vi "temperature_controller.vi"() -> ()   [LabVIEW 2017]
doc: "Use this template to build a simple state machine design pattern. Each state executes code and determines which state to transition to."
uses:
  controls/State.ctl
  <vilib>/Utility/error.llb/DialogType.ctl
  <instrlib>/LakeShore 336/Public/Data/Sensor Data (Single Reading).vi
  <instrlib>/LakeShore 336/Lake Shore 336.lvlib
panel:
  out "SetPoint":dbl format="%#_5f"
  out "Session Out":refnum<visa-resource-name>
  out "error out":errorcluster
  in  "Session In":refnum<visa-resource-name>="LakeShore336"
  in  "error in (no error)":errorcluster
  in  "SetPoint":dbl
  out "Heater percent":dbl
  in  "Heater":u16(ring) items=["Off", "Low", "Medium", "High"]
  out "Input A":dbl format="%#_5f"
  out "Input B":dbl format="%#_5f"
  in  "Exit Button":bool
  out "Status":string="Shutting down..."
  # "K"
  # "K"
  # "%"
  # "K"
  # "K"
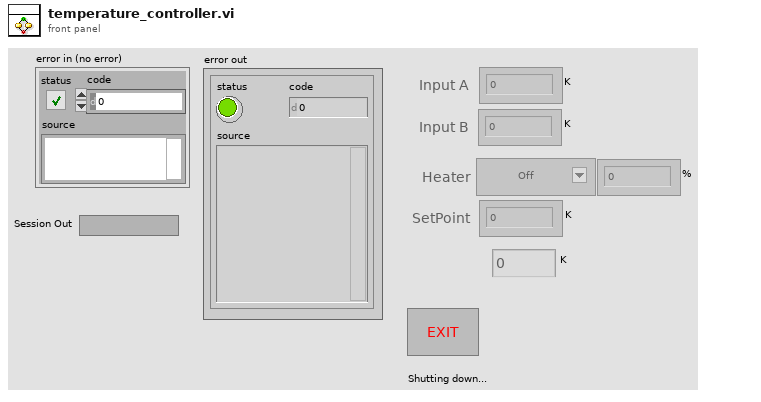
[diagram p1: front panel]
types:
  T1 = typedef "State.ctl" = enum16{"Init", "Idle", "Shutdown"}
  T2 = cluster{"Baud Rate":u32, "Parity":u16, "Data Bits":u16, "Stop Bits":u16, "Flow Control":u16}
  T3 = typedef "DialogType.ctl" = u16
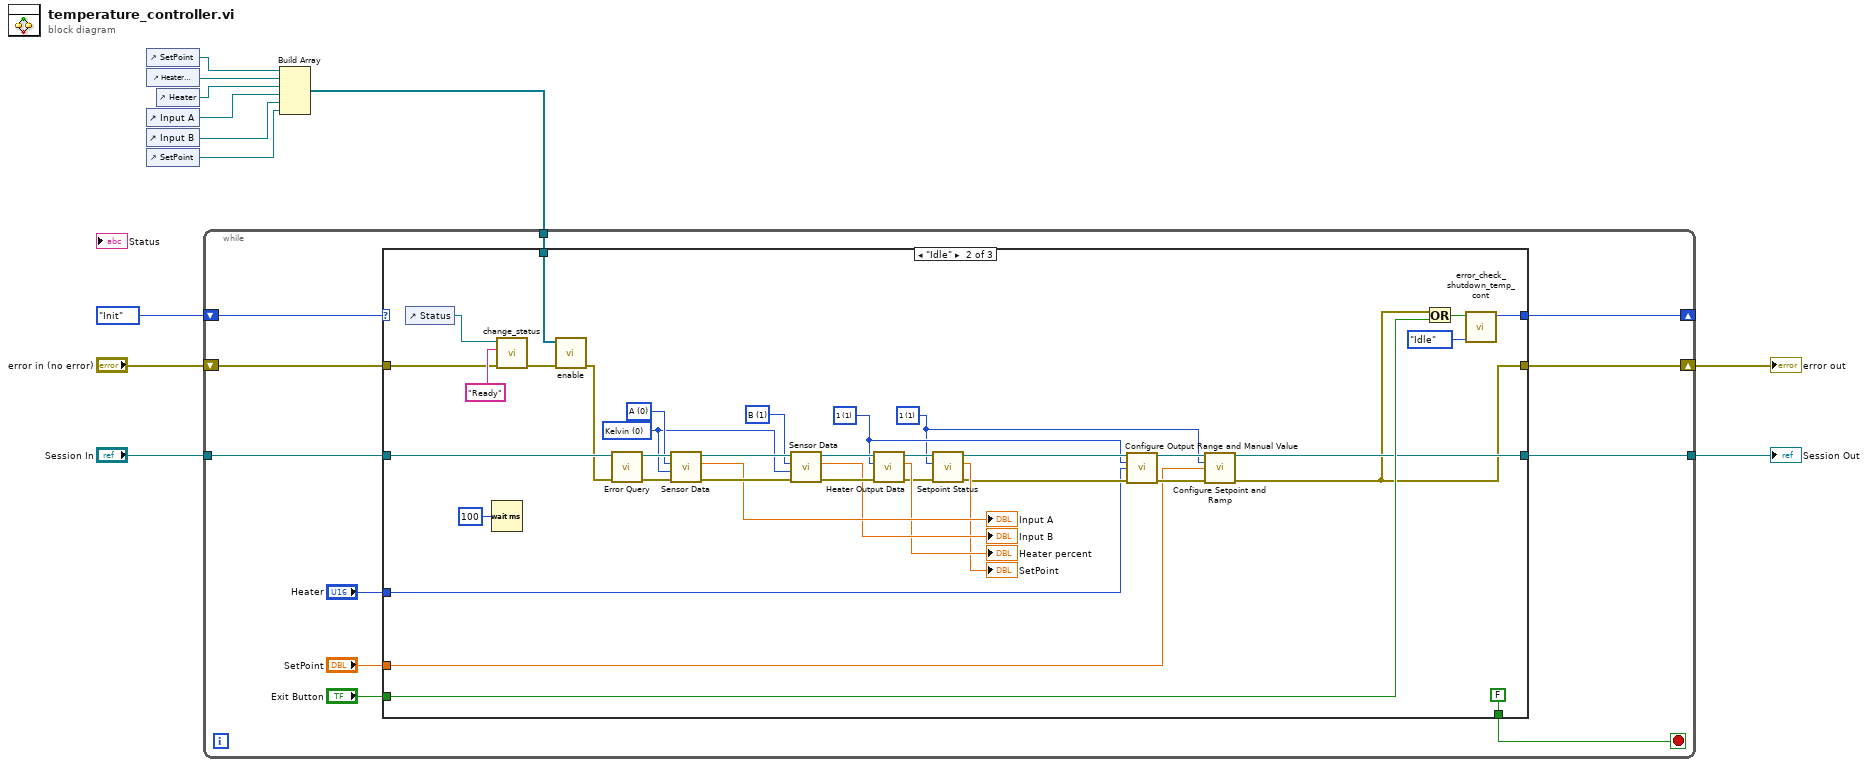
[diagram p0: block diagram]
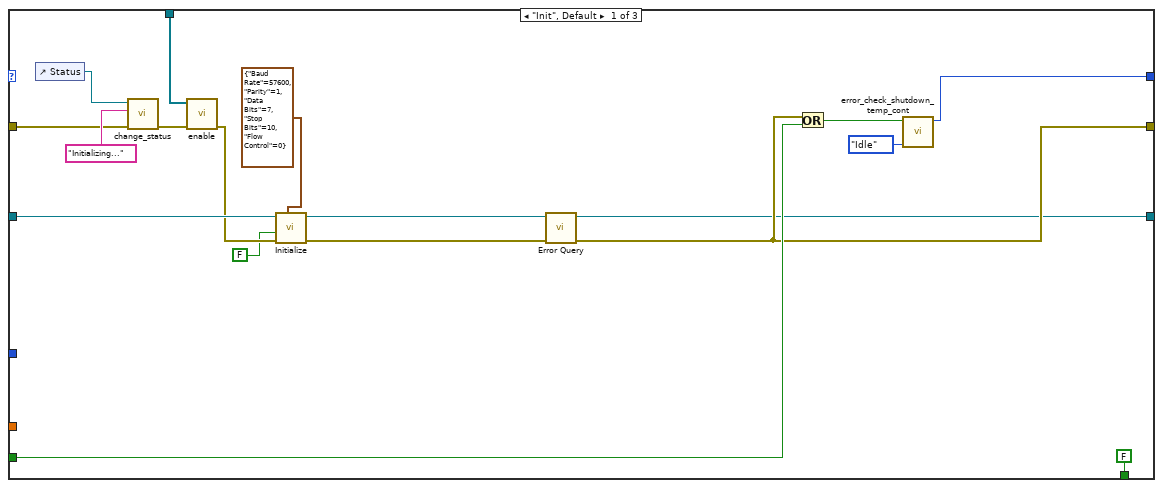
[diagram p2: hidden frame]
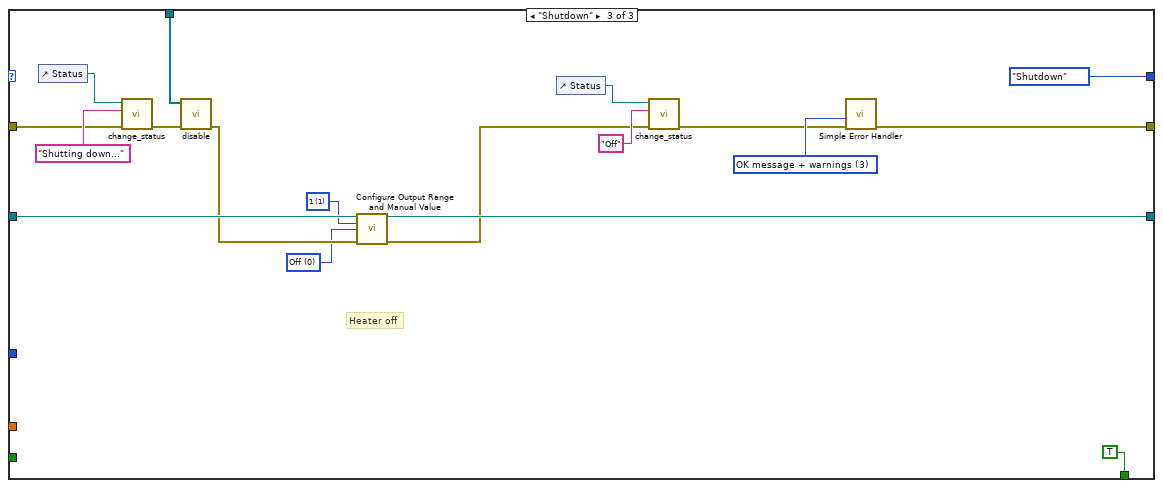
[diagram p3: hidden frame]
diagram:
  n1 = control-ref of="SetPoint"() -> (w12:refnum<vi>)
  n2 = control-ref of="Heater percent"() -> (w11:refnum<vi>)
  n3 = control-ref of="Input A"() -> (w9:refnum<vi>)
  n4 = control-ref of="Input B"() -> (w8:refnum<vi>)
  n5 = control-ref of="SetPoint"() -> (w1:refnum<vi>)
  n6 = control-ref of="Heater"() -> (w10:refnum<vi>)
  n7 = Build Array(w12, w11, w10, w9, w8, w1) -> (w7:refnum<vi>[])
  n8 = while {
    tunnel: w7 -> [w23]
    shift-right: [w18] -> _
    shift-left: State."Init" ("States") -> [w22]
    tunnel: "Session In" -> [w20]
    shift-right: [w19] -> w3
    shift-left: "error in (no error)" -> [w21]
    tunnel: [w14] -> w2
    stop <- w13 stop-if-true
    n9 = case shown="\"Idle\"" w22 {
      tunnel: w23 -> [w37 w79 w94]
      tunnel: w21 -> [w39 w75 w95]
      tunnel: w20 -> [w31 w68 w85]
      tunnel: [w29 w42 w92] -> w19
      tunnel: [w33 w71 State."Shutdown" ("s? t:f")] -> w18
      tunnel: "Exit Button" -> [w36 w72 _]
      tunnel: "Heater" -> [_ w48 _]
      tunnel: "SetPoint" -> [_ w44 _]
      tunnel: [w28 w45 w84] -> w14
      tunnel: [FALSE FALSE TRUE] -> w13
      frame "Init", Default {
        n10 = control-ref of="Status"() -> (w38:refnum<vi>)
        n11 = call "change_status.vi"("error in (no error)"=w39, "String"="Initializing...", "String in"=w38) -> ("error out"=w41:errorcluster)  [unwired: 8 in]
        n12 = call "enable.vi"("error in (no error)"=w41, "Array"=w37) -> ("error out"=w30:errorcluster)  [unwired: 9 in]
        n13 = call <instrlib>:"Initialize.vi"("Serial Configuration"=T2 {"Baud Rate"=57600, "Parity"=1, "Data Bits"=7, "Stop Bits"=10, "Flow Control"=0}, "error in (no error)"=w30, "Reset (True)"=FALSE, "VISA resource name"=w31) -> ("error out"=w24:errorcluster, "VISA resource name out"=w25:refnum<visa-resource-name>)  [unwired: 6 in]
        n14 = call <instrlib>:"Error Query.vi"("error in (no error)"=w24, "VISA resource name"=w25) -> ("error out"=w29:errorcluster, "VISA resource name out"=w28:refnum<visa-resource-name>)  [unwired: 7 in, 1 out]
        n15 = Or(x=w29, y=w36) -> (x .or. y?=w35:bool)
        n16 = call "error_check_shutdown_temp_cont.vi"("f"=State."Idle", "Boolean"=w35) -> ("s? t:f"=w33:T1)  [unwired: 9 in]
      }
      frame "Idle" {
        w43 = u16 1 items=["1"=1, "2"=2, "3"=3, "4"=4] ("Output (1:1)")
        w49 = u16 1 items=["1"=1, "2"=2] ("Heater Output (1:1)")
        w61 = u16 1 items=["A", "B", "C", "D"] ("Input (0:A)")
        w60 = u16 0 items=["Kelvin", "Celsius", "Sensor Units"] ("Data Source (0:Kelvin)")
        w64 = u16 0 items=["A", "B", "C", "D"] ("Input (0:A)")
        n17 = control-ref of="Status"() -> (w77:refnum<vi>)
        n18 = Wait (ms)(milliseconds to wait=u32 100) -> ()  [unwired: 1 out]
        n19 = call "change_status.vi"("error in (no error)"=w75, "String"="Ready", "String in"=w77) -> ("error out"=w78:errorcluster)  [unwired: 8 in]
        n20 = call "enable.vi"("error in (no error)"=w78, "Array"=w79) -> ("error out"=w67:errorcluster)  [unwired: 9 in]
        n21 = call <instrlib>:"Error Query.vi"("error in (no error)"=w67, "VISA resource name"=w68) -> ("error out"=w65:errorcluster, "VISA resource name out"=w66:refnum<visa-resource-name>)  [unwired: 7 in, 1 out]
        n22 = call-poly <instrlib>:"Sensor Data.vi"("error in (no error)"=w65, "Data Source (0:Kelvin)"=w60, "Input (0:A)"=w64, "VISA resource name"=w66) -> ("error out"=w62:errorcluster, "Sensor Data"=→"Input A":dbl, "VISA resource name out"=w63:refnum<visa-resource-name>)  [unwired: 5 in]
        n23 = call-poly <instrlib>:"Sensor Data.vi"("error in (no error)"=w62, "Data Source (0:Kelvin)"=w60, "Input (0:A)"=w61, "VISA resource name"=w63) -> ("error out"=w58:errorcluster, "Sensor Data"=→"Input B":dbl, "VISA resource name out"=w59:refnum<visa-resource-name>)  [unwired: 5 in]
        n24 = call <instrlib>:"Heater Output Data.vi"("error in (no error)"=w58, "Heater Output (1:1)"=w49, "VISA resource name"=w59) -> ("error out"=w53:errorcluster, "Output Value"=→"Heater percent":dbl, "VISA resource name out"=w54:refnum<visa-resource-name>)  [unwired: 6 in]
        n25 = call <instrlib>:"Setpoint Status.vi"("error in (no error)"=w53, "Output (1:1)"=w43, "VISA resource name"=w54) -> ("error out"=w50:errorcluster, "Setpoint"=→"SetPoint":dbl, "VISA resource name out"=w51:refnum<visa-resource-name>)  [unwired: 6 in]
        n26 = call <instrlib>:"Configure Output Range and Manual Value.vi"("VISA resource name"=w51, "Output (1:1)"=w49, "Range (0:Off)"=w48, "error in (no error)"=w50) -> ("VISA resource name out"=w47:refnum<visa-resource-name>, "error out"=w46:errorcluster)  [unwired: 10 in]
        n27 = call <instrlib>:"Configure Setpoint and Ramp.vi"("VISA resource name"=w47, "Output's Control Loop (1:1)"=w43, "Setpoint (0.00000)"=w44, "error in (no error)"=w46) -> ("VISA resource name out"=w45:refnum<visa-resource-name>, "error out"=w42:errorcluster)  [unwired: 10 in]
        n28 = Or(x=w42, y=w72) -> (x .or. y?=w74:bool)
        n29 = call "error_check_shutdown_temp_cont.vi"("f"=State."Idle", "Boolean"=w74) -> ("s? t:f"=w71:T1)  [unwired: 9 in]
      }
      frame "Shutdown" {
        w80 = u16 1 items=["1"=1, "2"=2, "3"=3, "4"=4] ("Output (1:1)")
        w81 = u16 0 items=["Off", "Low (On)", "Medium", "High"] ("Range (0:Off)")
        w91 = T3 3 items=["no dialog", "OK message", "continue or stop message", "OK message + warnings", "continue/stop + warnings"] ("type of dialog (OK msg:1)")
        # "Heater off"
        n30 = control-ref of="Status"() -> (w93:refnum<vi>)
        n31 = call "change_status.vi"("error in (no error)"=w95, "String"="Shutting down...", "String in"=w93) -> ("error out"=w97:errorcluster)  [unwired: 8 in]
        n32 = call "disable.vi"("error in (no error)"=w97, "Array"=w94) -> ("error out"=w83:errorcluster)  [unwired: 9 in]
        n33 = call <instrlib>:"Configure Output Range and Manual Value.vi"("VISA resource name"=w85, "Output (1:1)"=w80, "Range (0:Off)"=w81, "error in (no error)"=w83) -> ("VISA resource name out"=w84:refnum<visa-resource-name>, "error out"=w82:errorcluster)  [unwired: 10 in]
        n34 = control-ref of="Status"() -> (w87:refnum<vi>)
        n35 = call "change_status.vi"("error in (no error)"=w82, "String"="Off", "String in"=w87) -> ("error out"=w88:errorcluster)  [unwired: 8 in]
        n36 = call <vilib>:"Simple Error Handler.vi"("type of dialog (OK msg:1)"=w91, "error in (no error)"=w88) -> ("error out"=w92:errorcluster)  [unwired: 3 in, 4 out]
      }
    }
  }
  "error out" <- w3
  "Session Out" <- w2
